vi "Graphic_UI_Main.vi"(7 "Graphic UI Exit":refnum<user-event>, 11 "manager_daemon":refnum<class "manager_daemon.lvclass">) -> ()   [LabVIEW 2024]
uses:
  typedefs/volume.type.colors--cluster.ctl
  comic_manager/manager_daemon/manager_daemon.lvclass
  <vilib>/Utility/miscctls.llb/LVPositionTypeDef.ctl
  <vilib>/Utility/miscctls.llb/LVPoint32TypeDef.ctl
  CV_Shared_Library/volume.object--cluster.ctl
  CV_Shared_Library/volume.type--enum.ctl
  comic_manager/TypeDefs/issue.display--cluster.ctl
  typedefs/picture.data--cluster.ctl
  typedefs/filters--cluster.ctl
  comic_manager/manager_daemon/manager_daemon.lvclass/manager_daemon.ctl
  comic_manager/TypeDefs/graphic.filter--cluster.ctl
  <vilib>/addons/_JKI Toolkits/State Machine/_JKI_lib_State_Machine.llb/Select State(s)_err__jki_lib_state_machine.vi
  <vilib>/addons/_JKI Toolkits/State Machine/_JKI_lib_State_Machine.llb/Periodic Trigger__ogtk__JKI-SM__jki_lib_state_machine.vi
  CV_Shared_Library/CV_Shared_Library.lvlib
panel:
  in  "change volume types":bool
  in  "dest type":T1=enum."Reprint/Document" caption="Enum"
  in  "source type":T1=enum."One Shot" caption="Enum"
  in  "search string":string
  in  "publisher":u16(ring)
  in  "advanced filter":bool
  in  "Release Week":timestamp format="%<%x>T"
  out "filter dates":cluster{"start":timestamp, "end":timestamp}={"start"=timestamp(3328668000 s since 1904-01-01), "end"=timestamp(3785292000 s since 1904-01-01)} {"start" format="%<%x>T"; "end" format="%<%x>T"}
  in  "zoom filter":bool
  in  "generate report":bool
  in  "Show/Hide Issues":bool
  in  "clear title":bool
  in  "titles":string[](array[string])=["x-men"]
  in  "Show All Comics":bool
  in  "Volume Type":T2={"Ongoing"=TRUE, "Limited Series"=TRUE, "Annuals"=TRUE, "One Shots"=TRUE, "Reference/Reprints"=TRUE, "Digital"=TRUE}
  in  "Exit":bool
  in  "Legend":T3={"ongoing"=34559, "Limited Series"=35193, "Annuals"=16754450, "One Shots"=7566195, "Reprints"=16722176, "Digital"=49407}
  out "2D Picture":picture
  in  "Show Legend":bool=TRUE
  in  "Step Size":enum32{"Monthly", "Yearly"}(radio)
  in  "inc time":bool
  in  "dec time":bool
  in  "dec end":bool
  in  "dec start":bool
  in  "inc start":bool
  in  "inc end":bool
  in  "Plot End":timestamp=timestamp(3785292000 s since 1904-01-01) format="%<%x>T"
  in  "Plot Start":timestamp=timestamp(3318732000 s since 1904-01-01) format="%<%x>T"
  out "volume":string="uncanny x-men (1981)"
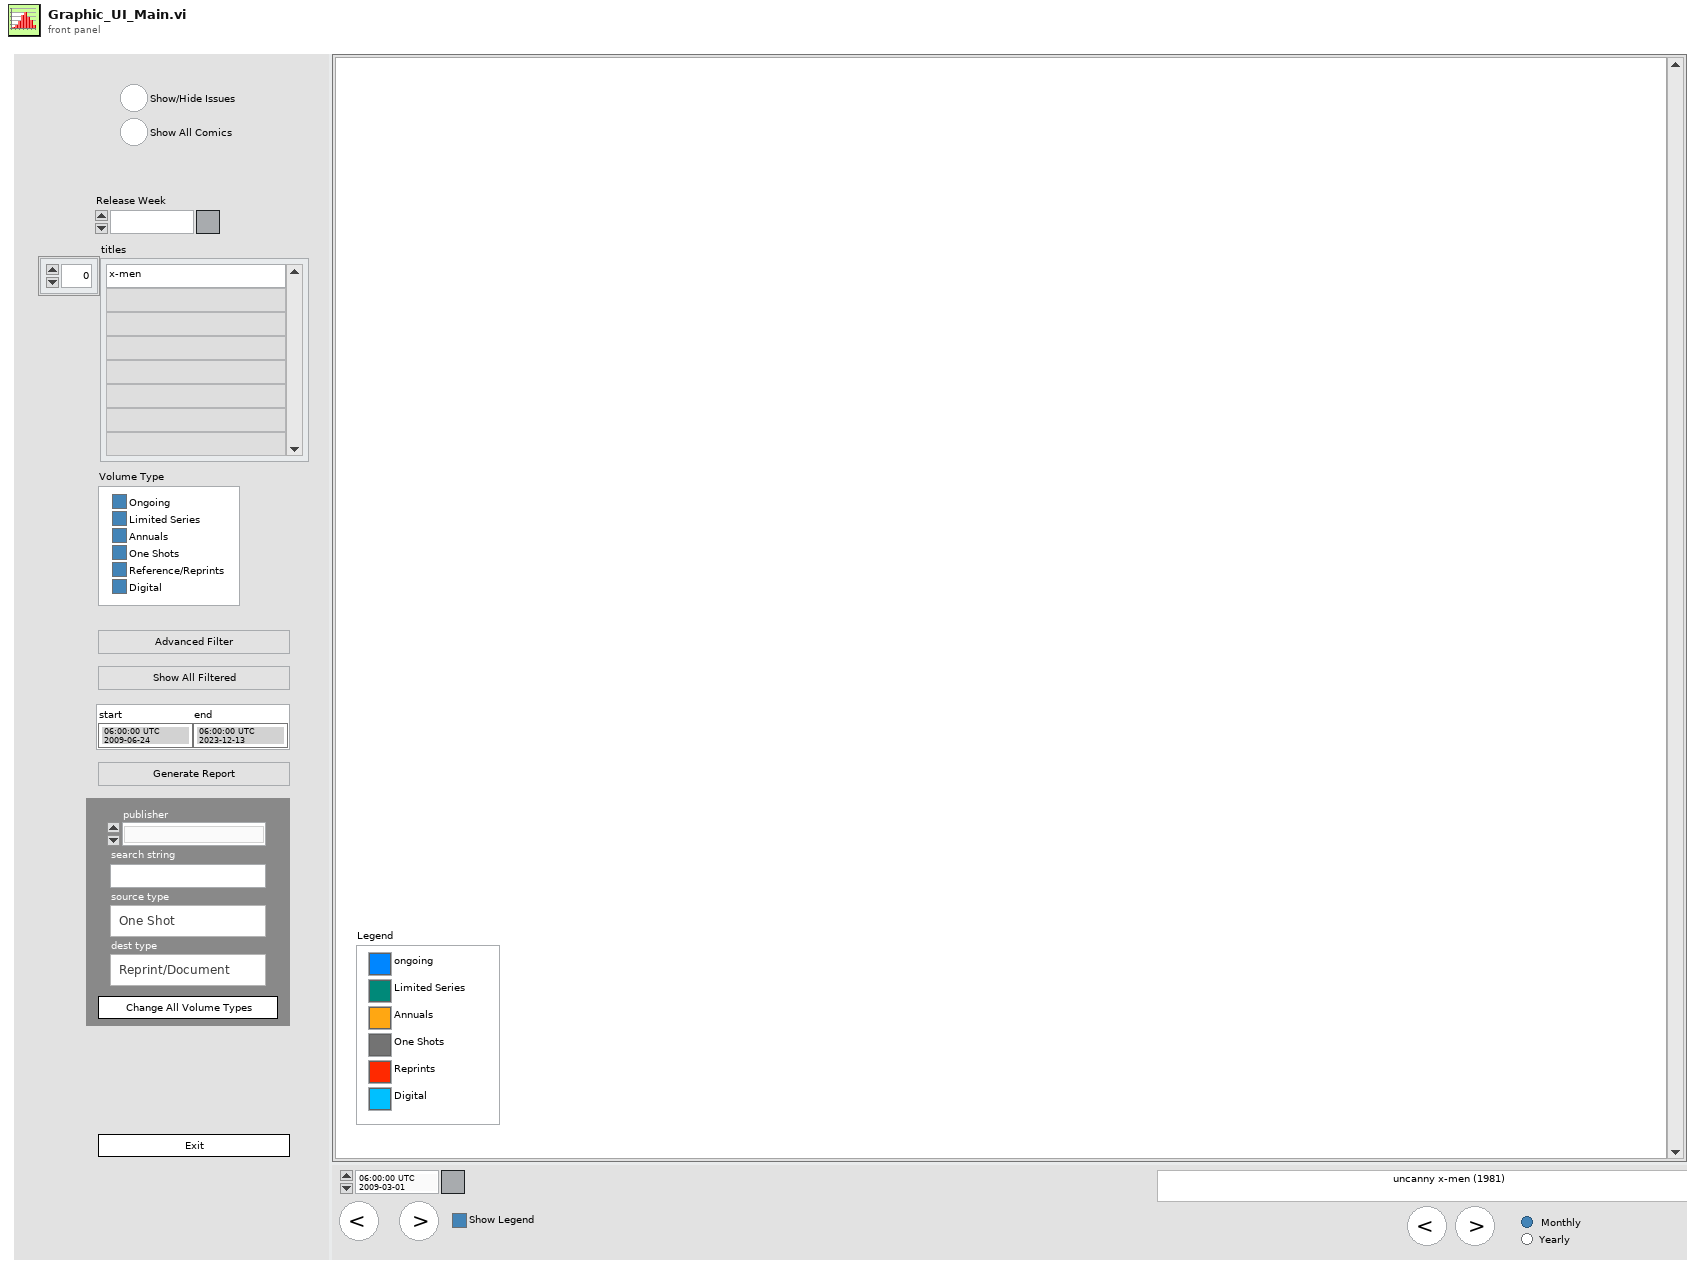
[diagram p1: front panel]
types:
  T1 = typedef "CV_Shared_Library.lvlib/volume.type--enum.ctl" = enum16{"Ongoing", "Limited Series", "Annual", "One Shot", "Reprint/Document", "Digital"}
  T2 = cluster{"Ongoing":bool, "Limited Series":bool, "Annuals":bool, "One Shots":bool, "Reference/Reprints":bool, "Digital":bool}
  T3 = typedef "volume.type.colors--cluster.ctl" = cluster{"ongoing":u32, "Limited Series":u32, "Annuals":u32, "One Shots":u32, "Reprints":u32, "Digital":u32}
  T4 = cluster{"search string":string, "source type":T1, "dest type":T1, "publisher":string}
  T5 = enum8{"Enabled", "Disabled", "Disabled and Grayed Out"}
  T6 = typedef "LVPositionTypeDef.ctl" = cluster{"Left":i32, "Top":i32}
  T7 = enum32{"Invalid", "Standard", "Closed", "Hidden", "Minimized", "Maximized"}
  T8 = enum32{"invalid app kind", "Development System", "Run Time System", "Student Edition", "Embedded LabVIEW", "Evaluation", "Custom"}
  T9 = typedef "filters--cluster.ctl" = cluster{"team filter":string[], "story filter":string[], "char filter":string[], "concept filter":string[], "Apply Filters":enum32{"AND", "OR"}}
  T10 = typedef "CV_Shared_Library.lvlib/graphic.filter--cluster.ctl" = cluster{"Volume Type":cluster{"Ongoing":bool, "Limited Series":bool, "Annuals":bool, "One Shots":bool, "Reference/Reprints":bool, "Digital":bool}, "team":string[], "characters":string[], "storyArcs":string[], "Plot End":timestamp, "Plot Start":timestamp, "title":string[], "colors":T3, "concept":string[], "show all":bool, "Search by Title":enum32{"AND", "OR"}, "pub ids":i32[]}
  T11 = cluster{"left":i16, "top":i16, "right":i16, "bottom":i16}
  T12 = typedef "CV_Shared_Library.lvlib/volume.object--cluster.ctl" = cluster{"start date":timestamp, "end date":timestamp, "sortable_name":string, "color":u32, "volume type":T1, "issues":T13[]}
  T13 = typedef "CV_Shared_Library.lvlib/issue.display--cluster.ctl" = cluster{"cover_date":timestamp, "id":i32, "number":string, "fill":bool, "hilight":bool}
  T14 = typedef "picture.data--cluster.ctl" = cluster{"names":string[], "colors":u32[], "cells":cluster{"left":i16, "top":i16, "right":i16, "bottom":i16}[], "end date":timestamp, "start date":timestamp}
  T15 = typedef "LVPoint32TypeDef.ctl" = cluster{"Horizontal":i32, "Vertical":i32}
  T16 = cluster{"Core":cluster{"Current VI Reference":refnum<vi>, "Close Panel on Exit?":bool}, "volume objects":cluster{"Array":T12[]}[], "picture data":T14, "picture":picture, "rows":cluster{"left":i16, "top":i16, "right":i16, "bottom":i16}[], "cursor":T15, "manager_daemon":refnum<class "manager_daemon.lvclass">, "filter dates":cluster{"start":timestamp, "end":timestamp}, "filters":T9, "pub filter event":refnum<user-event>, "pub ids":i32[], "filter event":refnum<user-event>, "Graphic UI Exit":refnum<user-event>, "filter exit":refnum<user-event>}
  T17 = typedef "manager_daemon.lvclass/PublisherMap--map.ctl" = map{string, T18}
  T18 = typedef "manager_daemon.lvclass/PublisherData--cluster.ctl" = cluster{"id":i32, "volumes":set{i32}}
  T19 = cluster{"left":i16, "top":i16, "right":i16, "bottom":i16}[]
  T20 = cluster{"Current VI Reference":refnum<vi>, "Close Panel on Exit?":bool}
  T21 = cluster{"filter data event":refnum<user-event>, "search titles event":refnum<user-event>}
  T22 = typedef "LVBoundsTypeDef.ctl" = cluster{"Width":u32, "Height":u32}
  T23 = typedef "LVPointTypeDef.ctl" = cluster{"Horizontal":i16, "Vertical":i16}
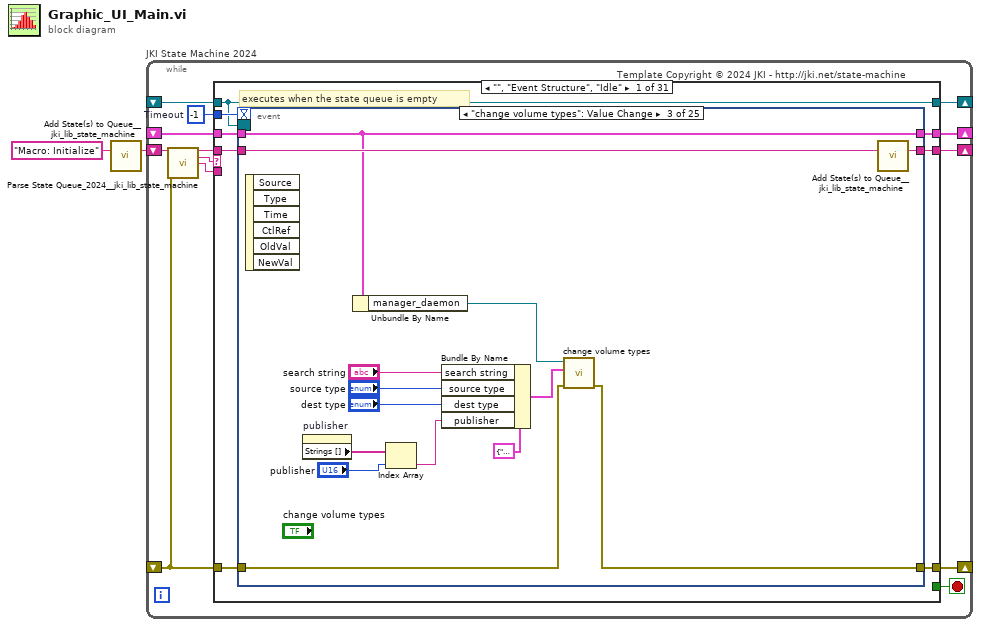
[diagram p0: block diagram]
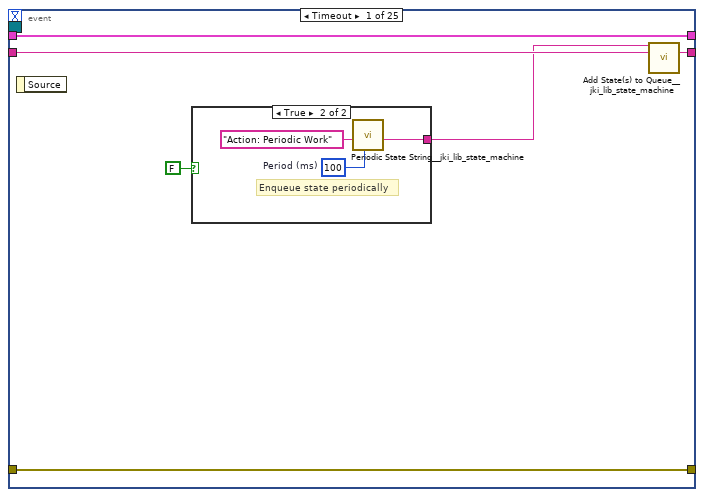
[diagram p2: hidden frame]
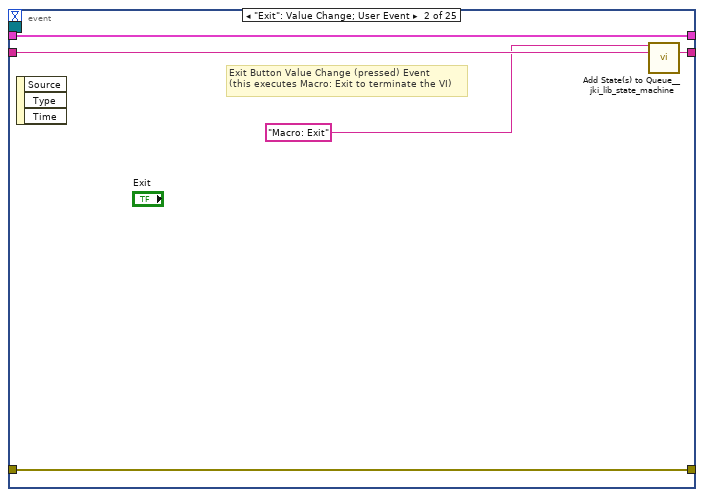
[diagram p4: hidden frame]
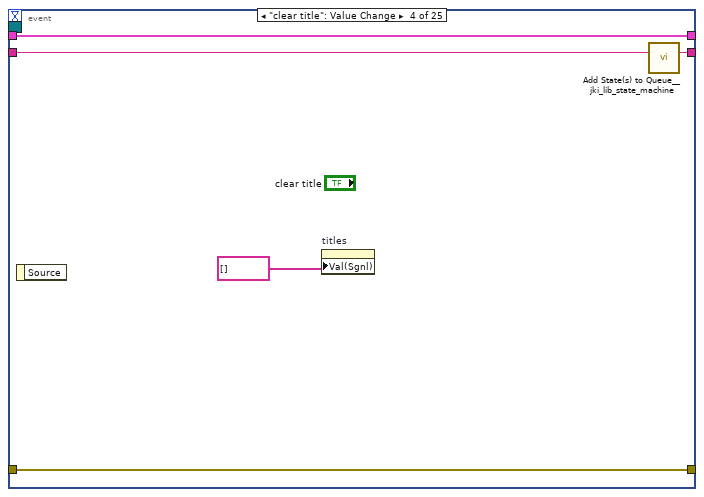
[diagram p5: hidden frame]
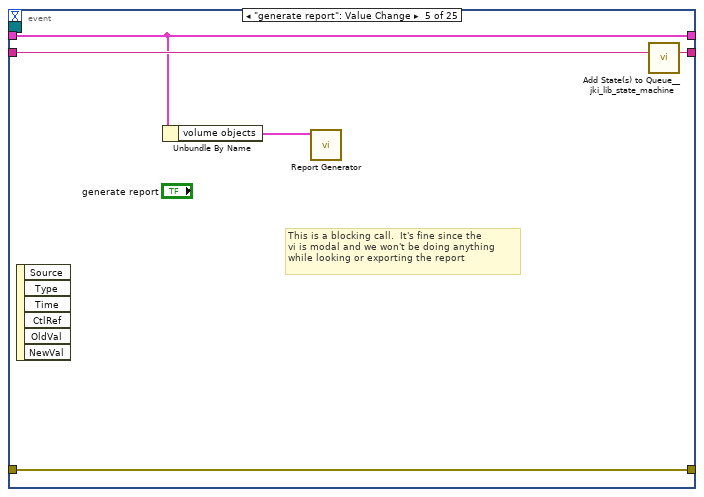
[diagram p6: hidden frame]
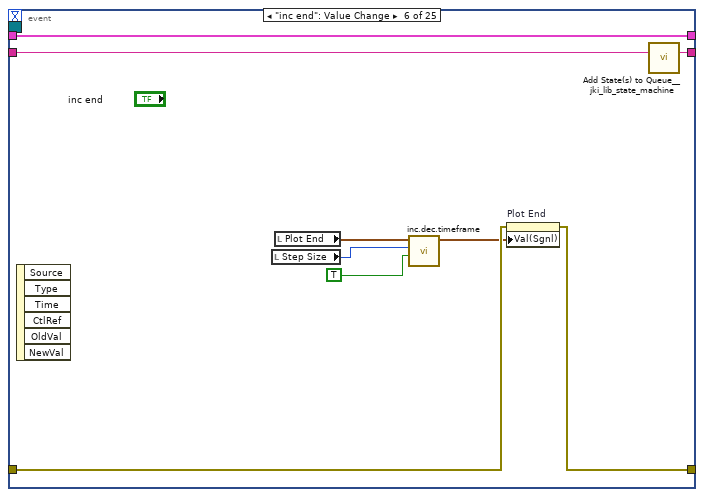
[diagram p7: hidden frame]
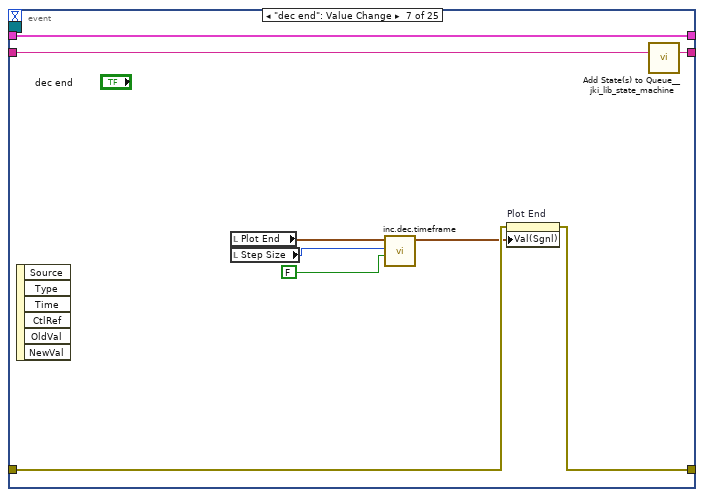
[diagram p8: hidden frame]
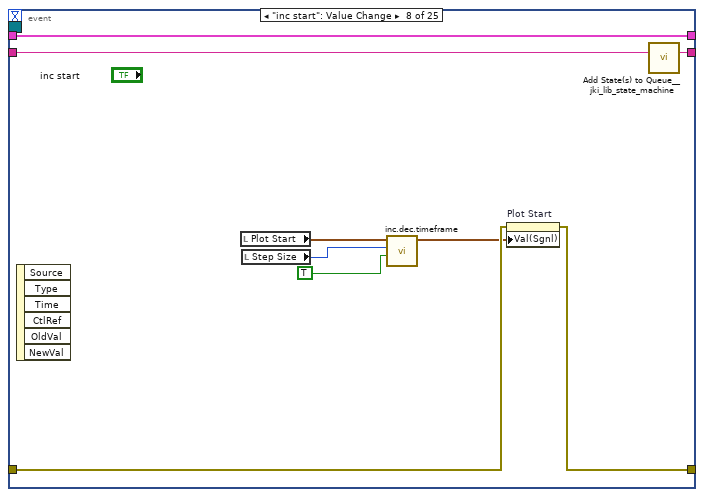
[diagram p9: hidden frame]
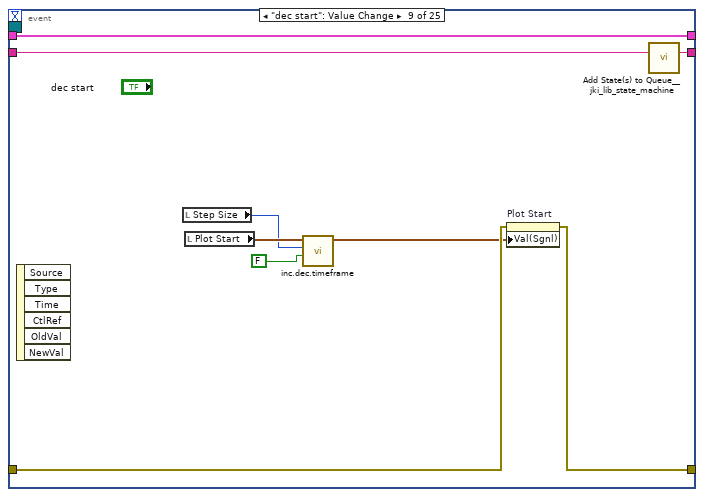
[diagram p10: hidden frame]
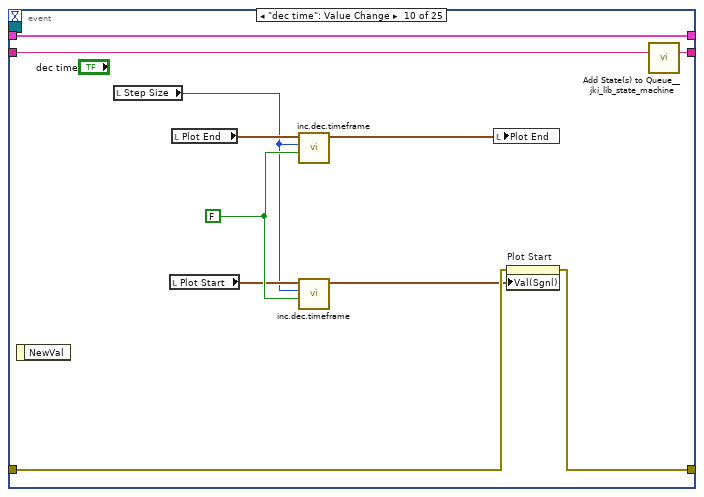
[diagram p11: hidden frame]
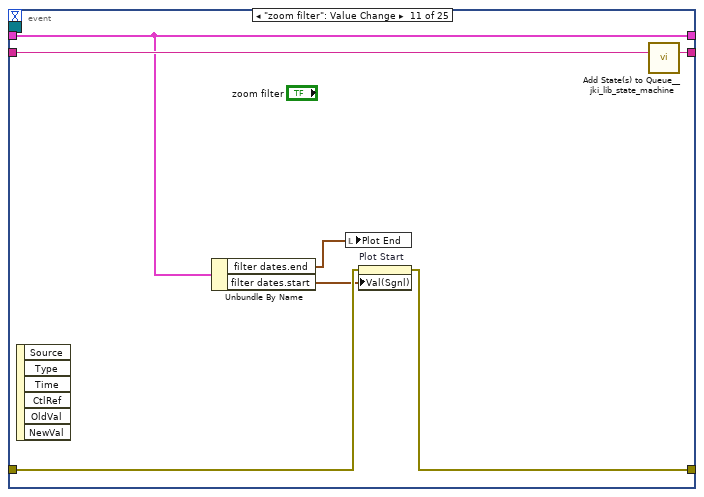
[diagram p12: hidden frame]
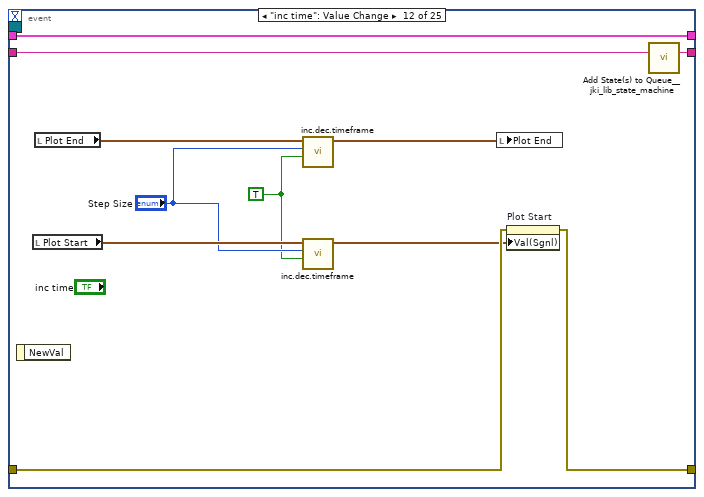
[diagram p13: hidden frame]
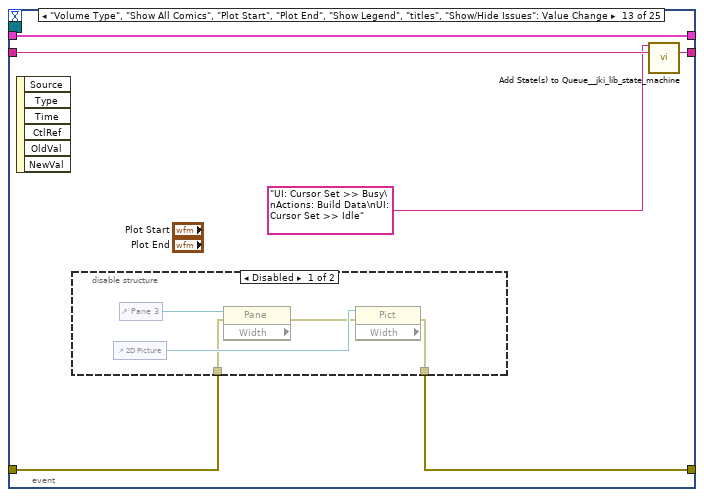
[diagram p14: hidden frame]
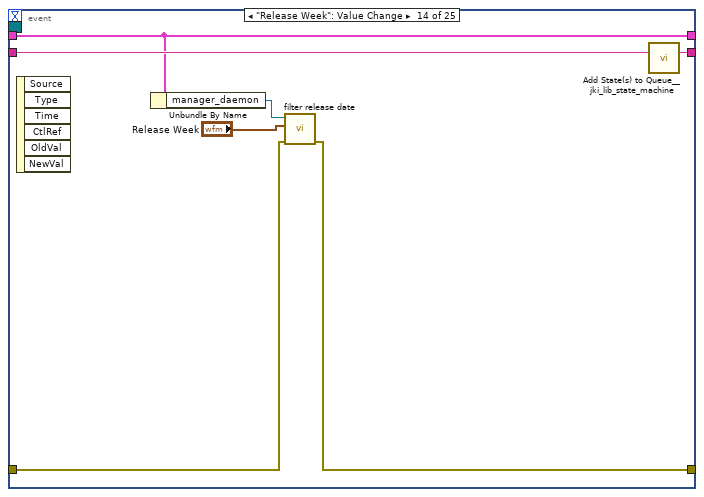
[diagram p16: hidden frame]
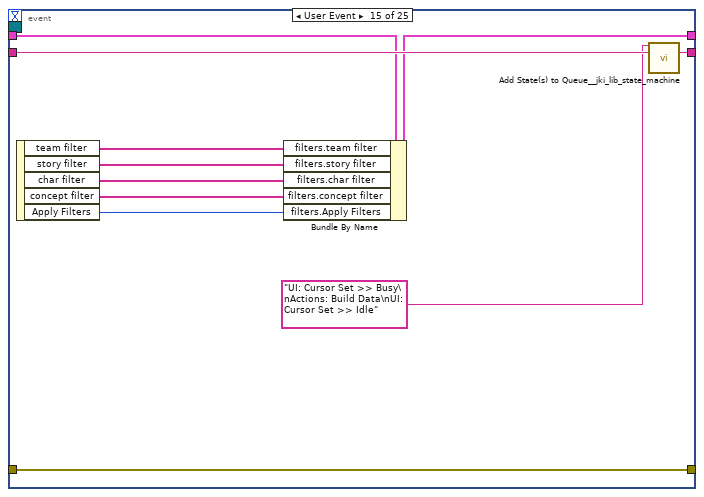
[diagram p17: hidden frame]
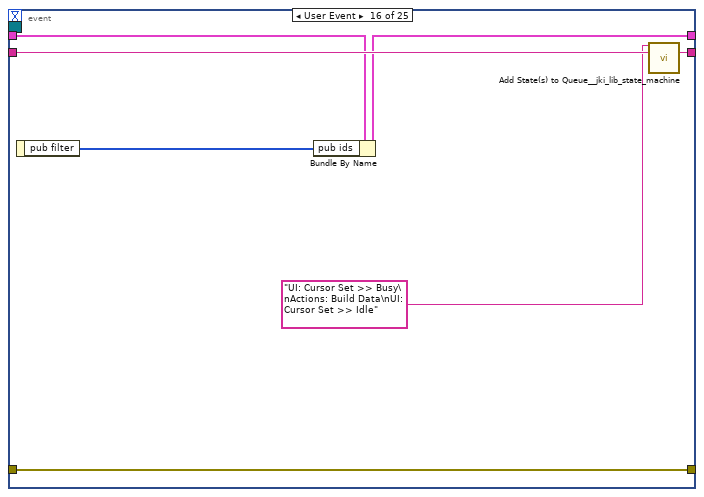
[diagram p18: hidden frame]
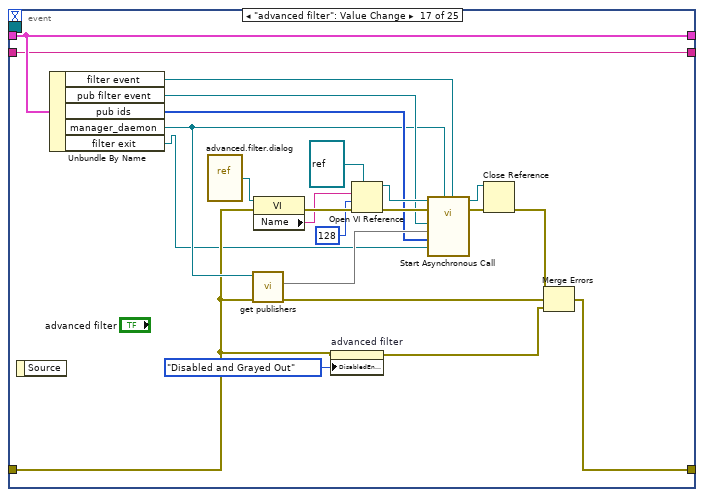
[diagram p19: hidden frame]
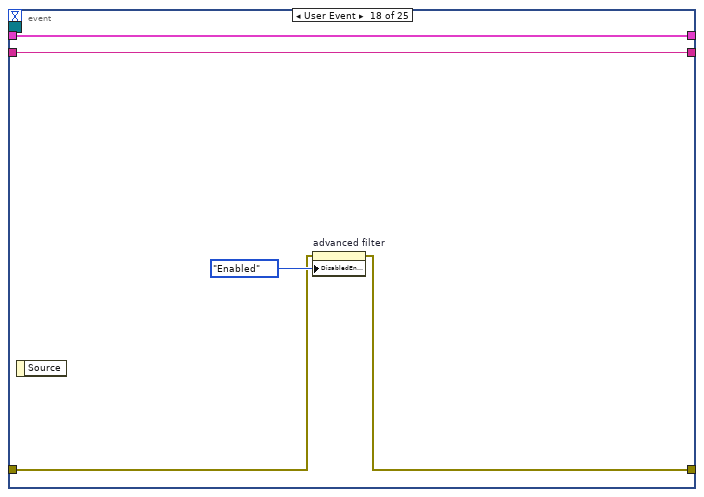
[diagram p20: hidden frame]
diagram:
  n1 = call <vilib>:"Add State(s) to Queue__jki_lib_state_machine.vi"("State(s) in (\"\")"="Macro: Initialize") -> ("States Out"=w2:string)  [unwired: 14 in]
  n2 = while "JKI State Machine 2024" {
    shift-right: [w8] -> _
    shift-left: _ -> [w7]
    shift-right: [w11] -> _
    shift-left: _ -> [w5]
    shift-right: [w10] -> _
    shift-left: w2 -> [w12]
    shift-right: [w4] -> _
    shift-left: _ -> [w3]
    stop <- w9 stop-if-true
    w6 = -1  # Timeout
    # "Template Copyright © 2024 JKI - http://jki.net/state-machine"
    n3 = call <vilib>:"Parse State Queue_2024__jki_lib_state_machine.vi"("State Queue"=w12, "Error In (no error)"=w5) -> ("Remaining States"=w14:string, "Current State"=w15:string, "Arguments"=w13:string)  [unwired: 11 in]
    n4 = case shown="\"\", \"Event Structure\", \"Idle\"" w15 {
      selector: w15 -> [_ _ w290 _ _ _ _ _ _ _ _ _ _ _ _ _ _ _ _ _ _ _ _ _ _ _ _ _ _ _ _]
      tunnel: w14 -> [w23 w288 w294 w314 w325 w335 w340 w359 w384 w389 w409 w415 w420 w430 w446 w454 w459 w466 w478 w548 w554 w564 w569 w579 w590 w602 w614 w633 w655 w669 w693]
      tunnel: w13 -> [_ _ _ _ w320 _ _ _ _ _ _ _ _ _ w442 _ _ w461 w472 _ _ _ _ _ _ _ _ _ _ _ _]
      tunnel: w7 -> [w21 w285 w292 w307 w322 w333 w337 _ w381 w386 w403 w413 w417 w427 w441 w452 w457 w464 w474 w545 w551 w562 w566 w573 w588 w600 w611 w631 w646 w663 w685]
      tunnel: [w20 w286 w296 w311 errorcluster {"status"=FALSE, "code"=0, "source"=""} ("error out") w332 w338 w356 w379 w387 w407 w410 w418 w421 w434 w451 w456 w462 w475 w546 w552 w559 w567 w571 w585 w597 w612 w628 w645 w667 w692] -> w11
      tunnel: w5 -> [w17 w286 w295 w311 w321 w332 w338 w356 w374 w387 w393 w411 w418 w425 w433 w451 w456 w463 w476 w546 w552 w559 w567 w575 w587 w599 w612 w629 w644 w667 w692]
      tunnel: [w22 w287 w293 w313 w324 w334 w339 w358 w383 w388 w408 w414 w419 w429 w445 w453 w458 w465 w477 w547 w553 w563 w568 w578 w589 w601 w613 w632 w654 w668 w693] -> w10
      tunnel: [_ _ _ _ _ TRUE _ _ _ _ _ _ _ _ _ _ _ _ _ _ _ _ _ _ _ _ _ _ _ _ _] -> w9
      tunnel: [w19 w285 w292 w312 w322 w333 w337 w357 w381 w386 w401 w413 w417 w427 w441 w452 w457 w464 w474 w545 w551 w562 w566 w570 w588 w595 w611 w631 w646 w662 w684] -> w8
      tunnel: w6 -> [w18 _ _ _ _ _ _ _ _ _ _ _ _ _ _ _ _ _ _ _ _ _ _ _ _ _ _ _ _ _ _]
      tunnel: [w16 w284 w289 w301 w315 w330 w336 w349 w380 w385 w394 w412 w416 w428 w444 w450 w455 w460 w471 w544 w549 w555 w565 w577 w582 w592 w603 w627 w648 w660 w680] -> w4
      tunnel: w3 -> [w16 w284 w289 w301 w315 w330 w336 w349 w380 w385 _ w412 w416 w428 w444 w450 w455 w460 w471 w544 w549 w555 w565 w577 w582 w592 w603 w627 w648 w660 w680]
      frame "", "Event Structure", "Idle" {
        # "executes when the state queue is empty"
        n5 = event shown="[2] \"change volume types\": Value Change" {
          selector: w16 -> [_ _ _ _ _ _ _ _ _ _ _ _ _ _ _ _ _ _ _ _ _ _ _ _ _]
          dyn-events: _ -> [_ _ _ _ _ _ _ _ _ _ _ _ _ _ _ _ _ _ _ _ _ _ _ _ _]
          timeout: w18 -> [_ _ _ _ _ _ _ _ _ _ _ _ _ _ _ _ _ _ _ _ _ _ _ _ _]
          tunnel: w23 -> [w29 w37 w51 w56 w61 w70 w79 w88 w97 w108 w115 w126 w132 w145 w156 w163 w177 w190 w201 w225 w229 w246 w263 w271 w283]
          tunnel: [w28 w36 w50 w55 w60 w69 w78 w87 w96 w107 w114 w125 w131 w144 w155 w162 w177 w190 w200 w224 w229 w245 w262 w270 w282] -> w22
          tunnel: w21 -> [w26 w34 w39 w53 w58 w68 w77 w86 w95 w106 w111 w124 w129 w143 w152 w159 w179 w191 w202 w222 w230 w244 w252 w268 w280]
          tunnel: [w27 w35 w48 w54 w59 w66 w75 w84 w93 w104 w112 w122 w127 w140 w154 w161 w170 w187 w199 w205 w226 w231 w261 w267 w281] -> w20
          tunnel: w17 -> [w27 w35 w49 w54 w59 w67 w76 w85 w94 w105 w113 w123 w128 w139 w154 w161 w167 w188 w199 w206 w227 w242 w261 w266 w281]
          tunnel: [w26 w34 w39 w53 w58 w68 w77 w86 w95 w106 w111 w124 w129 w143 w151 w158 w179 w191 w202 w221 w230 w244 w251 w268 w280] -> w19
          event Timeout {
            n6 = event-data() -> ()  [unwired: 1 in, 1 out]
            n7 = case shown="True" FALSE {
              tunnel: [_ w32] -> w25
              frame False {
              }
              frame True {
                w30 = u32 100  # Period (ms)
                # "Enqueue state periodically"
                n8 = call <vilib>:"Periodic State String__jki_lib_state_machine.vi"("Period (ms)"=w30, "State"="Action: Periodic Work") -> ("State Out"=w32:string)  [unwired: 9 in]
              }
            }
            n9 = call <vilib>:"Add State(s) to Queue__jki_lib_state_machine.vi"("State(s) in Front (\"\")"=w25, "State(s) in (\"\")"=w29) -> ("States Out"=w28:string)  [unwired: 13 in]
          }
          event "Exit": Value Change; User Event {
            # "Exit Button Value Change (pressed) Event\n(this executes Macro: Exit to terminate the VI)"
            n10 = event-data() -> ()  [unwired: 1 in, 3 out]
            n11 = call <vilib>:"Add State(s) to Queue__jki_lib_state_machine.vi"("State(s) in Front (\"\")"="Macro: Exit", "State(s) in (\"\")"=w37) -> ("States Out"=w36:string)  [unwired: 13 in]
          }
          event "change volume types": Value Change {
            n12 = event-data() -> ()  [unwired: 1 in, 6 out]
            n13 = property on="publisher" class="Ring (strict)"() -> ("Strings []"=w43:string[])  [unwired: 2 in, 2 out]
            n14 = Unbundle By Name(w39) -> ("manager_daemon"=w38:refnum<class "manager_daemon.lvclass">)
            n15 = Index Array(array=w43, index="publisher") -> (element=w41:string)
            n16 = Bundle By Name(cluster=T4 {"search string"="", "source type"=enum."Ongoing", "dest type"=enum."Ongoing", "publisher"=""} ("change criteria"), "search string"="search string", "source type"="source type", "dest type"="dest type", "publisher"=w41) -> (w40:T4)
            n17 = call "change volume types.vi"("error in (no error)"=w49, "change criteria"=w40, "manager_daemon in"=w38) -> ("error out"=w48:errorcluster)  [unwired: 7 in, 1 out]
            n18 = call <vilib>:"Add State(s) to Queue__jki_lib_state_machine.vi"("State(s) in (\"\")"=w51) -> ("States Out"=w50:string)  [unwired: 14 in]
          }
          event "clear title": Value Change {
            n19 = event-data() -> ()  [unwired: 1 in, 1 out]
            n20 = property on="titles" class="Arr (strict)"("Val(Sgnl)"=string[] []) -> ()  [unwired: 2 in, 2 out]
            n21 = call <vilib>:"Add State(s) to Queue__jki_lib_state_machine.vi"("State(s) in (\"\")"=w56) -> ("States Out"=w55:string)  [unwired: 14 in]
          }
          event "generate report": Value Change {
            # "This is a blocking call.  It's fine since the \nvi is modal and we won't be doing anything\nwhile looking or exporting the report"
            n22 = event-data() -> ()  [unwired: 1 in, 6 out]
            n23 = Unbundle By Name(w58) -> ("volume objects"=w57:cluster{"Array":T12[]}[])
            n24 = call "Report Generator.vi"("volume objects"=w57) -> ()  [unwired: 11 in]
            n25 = call <vilib>:"Add State(s) to Queue__jki_lib_state_machine.vi"("State(s) in (\"\")"=w61) -> ("States Out"=w60:string)  [unwired: 14 in]
          }
          event "inc end": Value Change {
            n26 = event-data() -> ()  [unwired: 1 in, 6 out]
            n27 = local read "Step Size"() -> (w63:enum32{"Monthly", "Yearly"})
            n28 = local read "Plot End"() -> (w65:timestamp)
            n29 = call "inc.dec.timeframe.vi"("inc (T)"=TRUE, "Step Size"=w63, "Plot End"=w65) -> ("time stamp"=w64:timestamp)  [unwired: 8 in]
            n30 = property on="Plot End" class="AbsTime (strict)"(error in=w67, "Val(Sgnl)"=w64) -> (error out=w66:errorcluster)  [unwired: 1 in, 1 out]
            n31 = call <vilib>:"Add State(s) to Queue__jki_lib_state_machine.vi"("State(s) in (\"\")"=w70) -> ("States Out"=w69:string)  [unwired: 14 in]
          }
          event "dec end": Value Change {
            n32 = event-data() -> ()  [unwired: 1 in, 6 out]
            n33 = local read "Plot End"() -> (w74:timestamp)
            n34 = local read "Step Size"() -> (w72:enum32{"Monthly", "Yearly"})
            n35 = call "inc.dec.timeframe.vi"("inc (T)"=FALSE, "Step Size"=w72, "Plot End"=w74) -> ("time stamp"=w73:timestamp)  [unwired: 8 in]
            n36 = property on="Plot End" class="AbsTime (strict)"(error in=w76, "Val(Sgnl)"=w73) -> (error out=w75:errorcluster)  [unwired: 1 in, 1 out]
            n37 = call <vilib>:"Add State(s) to Queue__jki_lib_state_machine.vi"("State(s) in (\"\")"=w79) -> ("States Out"=w78:string)  [unwired: 14 in]
          }
          event "inc start": Value Change {
            n38 = event-data() -> ()  [unwired: 1 in, 6 out]
            n39 = local read "Plot Start"() -> (w83:timestamp)
            n40 = local read "Step Size"() -> (w81:enum32{"Monthly", "Yearly"})
            n41 = call "inc.dec.timeframe.vi"("inc (T)"=TRUE, "Step Size"=w81, "Plot End"=w83) -> ("time stamp"=w82:timestamp)  [unwired: 8 in]
            n42 = property on="Plot Start" class="AbsTime (strict)"(error in=w85, "Val(Sgnl)"=w82) -> (error out=w84:errorcluster)  [unwired: 1 in, 1 out]
            n43 = call <vilib>:"Add State(s) to Queue__jki_lib_state_machine.vi"("State(s) in (\"\")"=w88) -> ("States Out"=w87:string)  [unwired: 14 in]
          }
          event "dec start": Value Change {
            n44 = event-data() -> ()  [unwired: 1 in, 6 out]
            n45 = local read "Step Size"() -> (w90:enum32{"Monthly", "Yearly"})
            n46 = local read "Plot Start"() -> (w92:timestamp)
            n47 = call "inc.dec.timeframe.vi"("inc (T)"=FALSE, "Step Size"=w90, "Plot End"=w92) -> ("time stamp"=w91:timestamp)  [unwired: 8 in]
            n48 = property on="Plot Start" class="AbsTime (strict)"(error in=w94, "Val(Sgnl)"=w91) -> (error out=w93:errorcluster)  [unwired: 1 in, 1 out]
            n49 = call <vilib>:"Add State(s) to Queue__jki_lib_state_machine.vi"("State(s) in (\"\")"=w97) -> ("States Out"=w96:string)  [unwired: 14 in]
          }
          event "dec time": Value Change {
            w101 = FALSE ("inc (T)")
            n50 = event-data() -> ()  [unwired: 1 in, 1 out]
            n51 = local read "Step Size"() -> (w98:enum32{"Monthly", "Yearly"})
            n52 = local read "Plot Start"() -> (w100:timestamp)
            n53 = local read "Plot End"() -> (w103:timestamp)
            n54 = call "inc.dec.timeframe.vi"("inc (T)"=w101, "Step Size"=w98, "Plot End"=w103) -> ("time stamp"=w102:timestamp)  [unwired: 8 in]
            n55 = call "inc.dec.timeframe.vi"("inc (T)"=w101, "Step Size"=w98, "Plot End"=w100) -> ("time stamp"=w99:timestamp)  [unwired: 8 in]
            n56 = local write "Plot End"(w102) -> ()
            n57 = property on="Plot Start" class="AbsTime (strict)"(error in=w105, "Val(Sgnl)"=w99) -> (error out=w104:errorcluster)  [unwired: 1 in, 1 out]
            n58 = call <vilib>:"Add State(s) to Queue__jki_lib_state_machine.vi"("State(s) in (\"\")"=w108) -> ("States Out"=w107:string)  [unwired: 14 in]
          }
          event "zoom filter": Value Change {
            n59 = event-data() -> ()  [unwired: 1 in, 6 out]
            n60 = Unbundle By Name(w111) -> ("filter dates.end"=w109:timestamp, "filter dates.start"=w110:timestamp)
            n61 = local write "Plot End"(w109) -> ()
            n62 = property on="Plot Start" class="AbsTime (strict)"(error in=w113, "Val(Sgnl)"=w110) -> (error out=w112:errorcluster)  [unwired: 1 in, 1 out]
            n63 = call <vilib>:"Add State(s) to Queue__jki_lib_state_machine.vi"("State(s) in (\"\")"=w115) -> ("States Out"=w114:string)  [unwired: 14 in]
          }
          event "inc time": Value Change {
            w116 = TRUE ("inc (T)")
            n64 = event-data() -> ()  [unwired: 1 in, 1 out]
            n65 = local read "Plot Start"() -> (w119:timestamp)
            n66 = local read "Plot End"() -> (w121:timestamp)
            n67 = call "inc.dec.timeframe.vi"("inc (T)"=w116, "Step Size"="Step Size", "Plot End"=w121) -> ("time stamp"=w120:timestamp)  [unwired: 8 in]
            n68 = call "inc.dec.timeframe.vi"("inc (T)"=w116, "Step Size"="Step Size", "Plot End"=w119) -> ("time stamp"=w118:timestamp)  [unwired: 8 in]
            n69 = local write "Plot End"(w120) -> ()
            n70 = property on="Plot Start" class="AbsTime (strict)"(error in=w123, "Val(Sgnl)"=w118) -> (error out=w122:errorcluster)  [unwired: 1 in, 1 out]
            n71 = call <vilib>:"Add State(s) to Queue__jki_lib_state_machine.vi"("State(s) in (\"\")"=w126) -> ("States Out"=w125:string)  [unwired: 14 in]
          }
          event "Volume Type", "Show All Comics", "Plot Start", "Plot End", "Show Legend", "titles", "Show/Hide Issues": Value Change {
            n72 = event-data() -> ()  [unwired: 1 in, 6 out]
            n73 = disable-structure shown="Disabled" {
              disable-tunnel: w128 -> [w134 w138]
              disable-tunnel: [w133 w138] -> w127
              frame Disabled {
                n74 = control-ref of="2D Picture"() -> (w136:refnum<vi>)
                n75 = control-ref of="Pane 3"() -> (w137:refnum<vi>)
                n76 = property class="Pane" props=["Width"](reference=w137, error in=w134) -> (error out=w135:errorcluster)  [unwired: 2 out]
                n77 = property class="Pict" props=["Width"](reference=w136, error in=w135) -> (error out=w133:errorcluster)  [unwired: 2 out]
              }
              frame Enabled {
              }
            }
            n78 = call <vilib>:"Add State(s) to Queue__jki_lib_state_machine.vi"("State(s) in Front (\"\")"="UI: Cursor Set >> Busy\nActions: Build Data\nUI: Cursor Set >> Idle", "State(s) in (\"\")"=w132) -> ("States Out"=w131:string)  [unwired: 13 in]
          }
          event "Release Week": Value Change {
            n79 = event-data() -> ()  [unwired: 1 in, 6 out]
            n80 = Unbundle By Name(w143) -> ("manager_daemon"=w142:refnum<class "manager_daemon.lvclass">)
            n81 = call "filter release date.vi"("error in (no error)"=w139, "Release Week"="Release Week", "manager_daemon in"=w142) -> ("error out"=w140:errorcluster)  [unwired: 7 in, 1 out]
            n82 = call <vilib>:"Add State(s) to Queue__jki_lib_state_machine.vi"("State(s) in (\"\")"=w145) -> ("States Out"=w144:string)  [unwired: 14 in]
          }
          event User Event {
            n83 = event-data() -> ("team filter"=w150:string[], "story filter"=w149:string[], "char filter"=w148:string[], "concept filter"=w147:string[], "Apply Filters"=w146:enum32{"AND", "OR"})  [unwired: 1 in]
            n84 = Bundle By Name(cluster=w152, "filters.team filter"=w150, "filters.story filter"=w149, "filters.char filter"=w148, "filters.concept filter"=w147, "filters.Apply Filters"=w146) -> (w151:T16)
            n85 = call <vilib>:"Add State(s) to Queue__jki_lib_state_machine.vi"("State(s) in Front (\"\")"="UI: Cursor Set >> Busy\nActions: Build Data\nUI: Cursor Set >> Idle", "State(s) in (\"\")"=w156) -> ("States Out"=w155:string)  [unwired: 13 in]
          }
          event User Event {
            n86 = event-data() -> ("pub filter"=w157:i32[])  [unwired: 1 in]
            n87 = Bundle By Name(cluster=w159, "pub ids"=w157) -> (w158:T16)
            n88 = call <vilib>:"Add State(s) to Queue__jki_lib_state_machine.vi"("State(s) in Front (\"\")"="UI: Cursor Set >> Busy\nActions: Build Data\nUI: Cursor Set >> Idle", "State(s) in (\"\")"=w163) -> ("States Out"=w162:string)  [unwired: 13 in]
          }
          event "advanced filter": Value Change {
            n89 = event-data() -> ()  [unwired: 1 in, 1 out]
            n90 = Unbundle By Name(w179) -> ("filter event"=w168:refnum<user-event>, "pub filter event"=w178:refnum<user-event>, "pub ids"=w173:i32[], "manager_daemon"=w169:refnum<class "manager_daemon.lvclass">, "filter exit"=w164:refnum<user-event>)
            n91 = vi-ref "advanced.filter.dialog.vi"() -> (w186:refnum<vi>)
            n92 = call "get publishers.vi"("error in (no error)"=w167, "manager_daemon in"=w169) -> ("error out"=w171:errorcluster, "Publisher Map"=w174:T17)  [unwired: 7 in, 1 out]
            n93 = property class="VI"(reference=w186, error in=w167) -> (error out=w185:errorcluster, "Name"=w183:string)  [unwired: 1 out]
            n94 = property on="advanced filter" class="Bool"(error in=w167, "DisabledEnum"=T5."Disabled and Grayed Out" ("Disabled")) -> (error out=w166:errorcluster)  [unwired: 1 in, 1 out]
            n95 = Open VI Reference(type specifier VI Refnum (for type only)=refnum<vi> refnum, vi path=w183, options=128, error in (no error)=w185) -> (vi reference=w180:refnum<vi>, error out=w181:errorcluster)  [unwired: 2 in]
            n96 = call-by-ref "Start Asynchronous Call"(reference=w180, error in=w181, "filters events"=w168, "manager_daemon"=w169, "filter exit event"=w164, "filtered publisher ids"=w173, "map"=w174, "pub filter event"=w178) -> (reference out=w175:refnum<vi>, error out=w176:errorcluster)  [unwired: 6 in]
            n97 = Close Reference(reference=w175, error in (no error)=w176) -> (error out=w172:errorcluster)
            n98 = Merge Errors(w172, w171, w166) -> (w170:errorcluster)
          }
          event User Event {
            n99 = event-data() -> ()  [unwired: 1 in, 1 out]
            n100 = property on="advanced filter" class="Bool"(error in=w188, "DisabledEnum"=T5."Enabled" ("Disabled")) -> (error out=w187:errorcluster)  [unwired: 1 in, 1 out]
          }
          event "2D Picture": Mouse Wheel {
            n101 = event-data() -> ("Orientation"=w198:enum16{"Horizontal", "Vertical"})  [unwired: 1 in]
            n102 = property on="2D Picture" class="Pict"() -> ("Top"=w196:i16)  [unwired: 2 in, 2 out]
            n103 = Equal?(x=w198, y=enum16{"Horizontal", "Vertical"}."Vertical") -> (x = y?=w195:bool)
            n104 = Greater Or Equal To 0?(x=w196) -> (x >= 0?=w194:bool)
            n105 = And(x=w195, y=w194) -> (x .and. y?=w193:bool)
            n106 = case shown="False" w193 {
              tunnel: [_ "UI: Cursor Set >> Busy\nActions: Build Data\nUI: Cursor Set >> Idle"] -> w192
              frame False {
                n107 = property on="2D Picture" class="Pict"("Top"=i16 0 ("Origin:Top")) -> ()  [unwired: 2 in, 2 out]
              }
              frame True {
              }
            }
            n108 = call <vilib>:"Add State(s) to Queue__jki_lib_state_machine.vi"("State(s) in Front (\"\")"=w192, "State(s) in (\"\")"=w201) -> ("States Out"=w200:string)  [unwired: 13 in]
          }
          event User Event {
            w213 = timestamp(0 s since 1904-01-01)
            n109 = event-data() -> ("filtered data"=w217:T12[], "filter dates"=w216:cluster{"start":timestamp, "end":timestamp})  [unwired: 1 in]
            "filter dates" <- w216
            n110 = Unbundle(w216) -> ("start"=w215:timestamp, "end"=w214:timestamp)
            n111 = Equal?(x=w213, y=w215) -> (x = y?=w212:bool)
            n112 = Equal?(x=w214, y=w213) -> (x = y?=w211:bool)
            n113 = call "sort.volumes.vi"("volumes"=w217) -> ("end date"=w218:timestamp, "start date"=w219:timestamp, "volumes by row"=w220:cluster{"Array":T12[]}[])  [unwired: 8 in]
            n114 = Or(x=w212, y=w211) -> (x .or. y?=w210:bool)
            n115 = Select(t=T5."Disabled and Grayed Out" ("Disabled"), s=w210, f=T5."Enabled" ("Disabled")) -> (s? t:f=w207:T5)
            n116 = Bundle By Name(cluster=w222, "volume objects"=w220, "picture data.start date"=w219, "picture data.end date"=w218, "filter dates"=w216) -> (w221:T16)
            n117 = property on="zoom filter" class="Bool"(error in=w206, "DisabledEnum"=w207) -> (error out=w205:errorcluster)  [unwired: 1 in, 1 out]
            n118 = call <vilib>:"Add State(s) to Queue__jki_lib_state_machine.vi"("State(s) in Front (\"\")"="UI: Cursor Set >> Busy\nUI: FP Update >> TRUE\nActions: Calculate Rows\nActions: Draw Grid\nActions: Calculate Cells\nActions: Draw Picture\nUI: FP Update >> FALSE\nUI: Cursor Set >> Idle", "State(s) in (\"\")"=w225) -> ("States Out"=w224:string)  [unwired: 13 in]
          }
          event User Event {
            n119 = event-data() -> ("titles"=w228:string[])  [unwired: 1 in]
            n120 = property on="titles" class="Arr (strict)"(error in=w227, "Val(Sgnl)"=w228) -> (error out=w226:errorcluster)  [unwired: 1 in, 1 out]
          }
          event Panel Resize {
            n121 = event-data() -> ("VIRef"=w243:refnum<vi>)  [unwired: 1 in]
            n122 = call "resize.navigation.pane.vi"("error in (no error)"=w242, "vi ref"=w243) -> ("error out"=w240:errorcluster)  [unwired: 9 in]
            n123 = invoke on="2D Picture" class="Pict" method="FitControlToPane"(error in=w240) -> (error out=w239:errorcluster)  [unwired: 2 in, 2 out]
            n124 = property on="2D Picture" class="Pict"(error in=w239) -> (error out=w232:errorcluster, "Height"=w236:u32)  [unwired: 1 in, 1 out]
            n125 = Subtract(x=w236, y=u32 259) -> (x-y=w234:u32)
            n126 = Bundle By Name(cluster=T6 {"Left"=0, "Top"=0} ("Position"), "Top"=w234, "Left"=24) -> (w233:T6)
            n127 = property on="Legend" class="Clust (strict)"(error in=w232, "Position"=w233) -> (error out=w231:errorcluster)  [unwired: 1 in, 1 out]
            n128 = call <vilib>:"Add State(s) to Queue__jki_lib_state_machine.vi"("State(s) in Front (\"\")"="UI: Cursor Set >> Busy\nActions: Build Data\nUI: Cursor Set >> Idle", "State(s) in (\"\")"=w246) -> ("States Out"=w245:string)  [unwired: 13 in]
          }
          event "2D Picture": Mouse Move {
            n129 = event-data() -> ("Coords"=w255:T15)  [unwired: 1 in]
            n130 = property on="2D Picture" class="Pict"() -> ("Position"=w260:T6, "Top"=w247:i16)  [unwired: 2 in, 2 out]
            n131 = Unbundle By Name(w255) -> ("Horizontal"=w259:i32, "Vertical"=w257:i32)
            n132 = Unbundle By Name(w260) -> ("Left"=w258:i32, "Top"=w256:i32)
            n133 = Subtract(x=w259, y=w258) -> (x-y=w254:i32)
            n134 = Subtract(x=w257, y=w256) -> (x-y=w249:i32)
            n135 = Add(x=w249, y=w247) -> (x+y=w248:i32)
            n136 = Bundle By Name(cluster=w255, "Horizontal"=w254, "Vertical"=w248) -> (w250:T15)
            n137 = Bundle By Name(cluster=w252, "cursor"=w250) -> (w251:T16)
            n138 = call <vilib>:"Add State(s) to Queue__jki_lib_state_machine.vi"("State(s) in Front (\"\")"="Actions: Display Cursor" ("State(s) in Front (\"\")"), "State(s) in (\"\")"=w263) -> ("States Out"=w262:string)  [unwired: 13 in]
          }
          event "2D Picture": Mouse Down? {
            n139 = event-data() -> ("Coords"=w269:T15, "Mods.Double Click"=w264:bool)  [unwired: 1 in]
            n140 = case shown="True" w264 {
              tunnel: w269 -> [_ _]
              tunnel: w268 -> [_ w277]
              tunnel: w266 -> [w272 w274]
              tunnel: [w272 w273] -> w267
              frame False {
              }
              frame True {
                n141 = Unbundle By Name(w277) -> ("manager_daemon"=w276:refnum<class "manager_daemon.lvclass">)
                n142 = local read "volume"() -> (w275:string)
                n143 = call "display info.vi"("error in (no error)"=w274, "volume name"=w275, "manager_daemon in"=w276) -> ("error out"=w273:errorcluster)  [unwired: 7 in, 1 out]
              }
            }
            n144 = event-data("Discard?"=TRUE) -> ()  [unwired: 4 in, 1 out]
            n145 = call <vilib>:"Add State(s) to Queue__jki_lib_state_machine.vi"("State(s) in (\"\")"=w271) -> ("States Out"=w270:string)  [unwired: 14 in]
          }
          event Panel Close? {
            # "Discard the event because we'll close the front panel ourselves in Macro: Exit"
            # "Close Panel button (pressed) Event\n(this executes Macro: Exit to terminate the VI)"
            n146 = event-data() -> ()  [unwired: 1 in, 1 out]
            n147 = event-data("Discard?"=TRUE) -> ()  [unwired: 1 in, 1 out]
            n148 = call <vilib>:"Add State(s) to Queue__jki_lib_state_machine.vi"("State(s) in Front (\"\")"="Macro: Exit", "State(s) in (\"\")"=w283) -> ("States Out"=w282:string)  [unwired: 13 in]
          }
        }
      }
      frame "---------- Core ----------" {
        # "Do not put any code in this frame.\n(it is a separator no-op)"
        n149 = call <vilib>:"Add State(s) to Queue__jki_lib_state_machine.vi"("State(s) in (\"\")"=w288) -> ("States Out"=w287:string)  [unwired: 14 in]
      }
      frame Default {
        w299 = 42 items=["No error", "Argument error", "Memory is full", "Out of zone", "End of file", "File already open", "Generic file I/O error", "File not found", "File permission error", "Disk is full", "Duplicate path", "Too many files open", "System feature not enabled", "Resource file not found", "Cannot add resource", "Resource not found", "Image not found", "Image memory error", "Pen does not exist", "Config type invalid", "Config token not found", "Config parse error", "Config memory error", "Bad external code format", "Bad external code offset", "External code not present", "Null window", "Destroy window error", "Null menu", "Print aborted", "Bad print record", "Print driver error", "Windows error during printing", "Memory error during printing", "Print dialog error", "Generic print error", "Invalid device refnum", "Device not found", "Device parameter error", "Device unit error", "Cannot open device", "Device call aborted", "Generic error", "Cancelled by user", "Object ID too low", "Object ID too high", "Object not in heap", "Unknown heap", "Unknown object (invalid DefProc)", "Unknown object (DefProc not in table)", "Message out of range", "Invalid (null) method", "Unknown message", "Manager call not supported", "Bad address", "Network operation in progress", "Network operation timed out", "Connection is busy", "Network attribute not supported", "Network error", "Address in use", "System out of memory", "Connection aborted", "Connection refused", "Not connected", "Already connected", "Connection closed", "Initialization error (interapplication manager)", "Bad occurrence", "Wait on unbound occurrence handler", "Occurrence queue overflow", "Datalog type conflict", "Unused", "Unrecognized type (interapplication manager)", "Memory corrupt", "Failed to make temporary DLL", "Old CIN version", "Drag socket not found", "Failed to load drop-object", "Failed to register OLE object", "Failed to release OLE object", "Format specifier type mismatch", "Unknown format specifier", "Too few format specifiers", "Too many format specifiers", "Scan failed", "Newer CIN version", "Error converting to variant", "Runtime menu error", "Password tampered", "Variant attribute not found", "Incompatible variant data type", "Event data is not available", "Event Store is not present", "Occurrence is not found", "Event Queue is not created", "Event info is not available", "Refnum passed is NULL", "Error retrieving Class GUID", "Error retrieving CoClass GUID", "Error retrieving TypeLib GUID.", "Bad built application magic bytes.", "Specific driver is different from the specific driver associated with the Logical Name.", "There is no session opened to the class driver.", "Max Error", "MAX - Error with config objects", "MAX - Error loading configuration", "MAX - Group not supported"]
        # "Current State"
        # "Do not delete, rename, or modify this frame.\n(this is used to capture unhandled states and typos)"
        # "Handle mistyped state name (developer tool)"
        n150 = Format Into String(format string="Software Exception: Unhandled State \"%s\"." ("message"), error in=w295, w290) -> (resulting string=w298:string, error out=w297:errorcluster)  [unwired: 1 in]
        n151 = call <vilib>:"Error Cluster From Error Code.vi"("show call chain? (False)"=TRUE, "error in (no error)"=w297, "error message (\"\")"=w298, "error code (0)"=w299) -> ("error out"=w296:errorcluster)  [unwired: 5 in]
        n152 = call <vilib>:"Add State(s) to Queue__jki_lib_state_machine.vi"("State(s) in (\"\")"=w294) -> ("States Out"=w293:string)  [unwired: 14 in]
      }
      frame "Initialize Core Data" {
        # "Do not delete, rename, or modify this frame.\n(this is used to determine panel behavior on exit)"
        # "originally closed?"
        # "exe?"
        # "If panel starts closed or is an EXE, then close it when we exit"
        n153 = property class="VI"() -> ("FP.State"=w304:T7)  [unwired: 2 in, 2 out]
        n154 = property class="App"() -> ("App.Kind"=w310:T8)  [unwired: 2 in, 2 out]
        n155 = control-ref of="Current VI Reference"() -> (w305:refnum<vi>)
        n156 = Equal?(x=w304, y=T7."Closed" ("Front Panel Window:State")) -> (x = y?=w302:bool)
        n157 = Equal?(x=w310, y=T8."Run Time System" ("Application:Kind")) -> (x = y?=w308:bool)
        n158 = Or(x=w302, y=w308) -> (x .or. y?=w306:bool)
        n159 = Bundle By Name(cluster=w307, "Core.Current VI Reference"=w305, "Core.Close Panel on Exit?"=w306) -> (w312:T16)
        n160 = call <vilib>:"Add State(s) to Queue__jki_lib_state_machine.vi"("State(s) in (\"\")"=w314) -> ("States Out"=w313:string)  [unwired: 14 in]
      }
      frame "Error Handler" {
        # "When running as sourcecode, this function will add previous state data to the error message to aid the developer in troubleshoot errors.\nIf run as an executable, no additional information is added to the error message."
        # "This state receives both Errors and Warnings which is how the Status of this wire can be FALSE"
        # "Unhandled Error -- Display it"
        # "Handle any errors or warnings here.\nYou can also output any states to clean-up after errors or warnings occur"
        # "Clear error or warning"
        n161 = disable-structure shown="Default" {
          disable-tunnel: w321 -> [w328 w329]
          disable-tunnel: w320 -> [w327 _]
          disable-tunnel: [w326 w329] -> w319
          frame condition #0 (active) {
            n162 = call <vilib>:"Append Error Details__jki_lib_state_machine.vi"("error in (no error)"=w328, "Previous State and Argument(s)"=w327) -> ("error out"=w326:errorcluster)  [unwired: 9 in]
          }
          frame condition #1 {
          }
        }
        n163 = call <vilib>:"General Error Handler.vi"("error in (no error)"=w319) -> ()  [unwired: 10 in, 5 out]
        n164 = call-poly <vilib>:"Select State(s)__jki_lib_state_machine.vi"("State(s) if True (\"\")"="/* Post Error States", "Select"=w319, "State(s) if False (\"\")"="/* Post Warning States") -> ("States Out"=w317:string)  [unwired: 12 in]
        n165 = call <vilib>:"Add State(s) to Queue__jki_lib_state_machine.vi"("State(s) in Front (\"\")"=w317, "State(s) in (\"\")"=w325) -> ("States Out"=w324:string)  [unwired: 13 in]
      }
      frame "Exit" {
        # "Do not put any code in this frame.\n(No errors that occur here will be handled.)"
        n166 = call <vilib>:"Add State(s) to Queue__jki_lib_state_machine.vi"("State(s) in (\"\")"=w335) -> ("States Out"=w334:string)  [unwired: 14 in]
      }
      frame "---------- Data ----------" {
        # "Do not put any code in this frame.\n(It is a separator no-op. You can make a copy of this frame to create a new Data frame)"
        n167 = call <vilib>:"Add State(s) to Queue__jki_lib_state_machine.vi"("State(s) in (\"\")"=w340) -> ("States Out"=w339:string)  [unwired: 14 in]
      }
      frame "Data: Initialize" {
        w341 = refnum<user-event> refnum  # filter exit
        w343 = T9 {"team filter"=[], "story filter"=[], "char filter"=[], "concept filter"=[], "Apply Filters"=enum."AND"}  # filters
        w344 = refnum<user-event> refnum  # filter event
        w345 = i32[] []  # pub ids
        w346 = refnum<user-event> refnum  # pub filter event
        w347 = cluster{"start":timestamp, "end":timestamp} {"start"=timestamp(0 s since 1904-01-01), "end"=timestamp(0 s since 1904-01-01)}  # filter dates
        w350 = T14 {"names"=[], "colors"=[], "cells"=[], "end date"=timestamp(0 s since 1904-01-01), "start date"=timestamp(0 s since 1904-01-01)}  # picture data
        w351 = cluster{"Array":T12[]}[] []  # volume objects
        w352 = T15 {"Horizontal"=0, "Vertical"=0}  # cursor
        w353 = T19 []  # rows
        w354 = picture data[5B]  # picture
        w355 = T20 {"Current VI Reference"=refnum, "Close Panel on Exit?"=FALSE}  # Core
        # "Data names and types of shift register data are defined by this bundle."
        # "Initialize the shift-register data, here.\n(data names are defined by what you wire into the bundle function)"
        n168 = Bundle("Core"=w355, "volume objects"=w351, "picture data"=w350, "picture"=w354, "rows"=w353, "cursor"=w352, "manager_daemon"="manager_daemon", "filter dates"=w347, "filters"=w343, "pub filter event"=w346, "pub ids"=w345, "filter event"=w344, "Graphic UI Exit"="Graphic UI Exit", "filter exit"=w341) -> (w357:T16)  [unwired: 1 in]
        n169 = call <vilib>:"Add State(s) to Queue__jki_lib_state_machine.vi"("State(s) in (\"\")"=w359) -> ("States Out"=w358:string)  [unwired: 14 in]
      }
      frame "Data: Cleanup" {
        # "Cleanup any data and references, here.\n(this is called automatically, by the Macro: Exit)"
        n170 = Unbundle By Name(w381) -> ("filter event"=w375:refnum<user-event>, "pub filter event"=w377:refnum<user-event>, "Core.Current VI Reference"=w382:refnum<vi>, "Graphic UI Exit"=w372:refnum<user-event>, "filter exit"=w364:refnum<user-event>)
        n171 = Generate User Event(user event=w372, event data cluster=TRUE ("event data")) -> (error out=w370:errorcluster)  [unwired: 2 in, 1 out]
        n172 = Generate User Event(user event=w364, event data cluster=TRUE ("event data")) -> (user event out=w363:refnum<user-event>, error out=w366:errorcluster)  [unwired: 2 in]
        n173 = Close Reference(reference=w382) -> (error out=w378:errorcluster)  [unwired: 1 in]
        n174 = call <vilib>:"Clear Errors.vi"("error in (no error)"=w370, "specific error code to clear (0: all)"=1) -> ("error out"=w368:errorcluster)  [unwired: 4 in, 1 out]
        n175 = call <vilib>:"Clear Errors.vi"("error in (no error)"=w366, "specific error code to clear (0: all)"=1) -> ("error out"=w362:errorcluster)  [unwired: 4 in, 1 out]
        n176 = Destroy User Event(user event=w377) -> (error out=w376:errorcluster)  [unwired: 1 in]
        n177 = Destroy User Event(user event=w375) -> (error out=w373:errorcluster)  [unwired: 1 in]
        n178 = Destroy User Event(user event=w363, error in=w362) -> (error out=w361:errorcluster)
        n179 = call <vilib>:"Clear Errors.vi"("error in (no error)"=w361) -> ("error out"=w360:errorcluster)  [unwired: 5 in, 1 out]
        n180 = Merge Errors(w374, w373, w376, w378, w368, w360) -> (w379:errorcluster)
        n181 = call <vilib>:"Add State(s) to Queue__jki_lib_state_machine.vi"("State(s) in (\"\")"=w384) -> ("States Out"=w383:string)  [unwired: 14 in]
      }
      frame "---------- Events ----------" {
        # "Do not put any code in this frame.\n(It is a separator no-op. You can make a copy of this frame to create a new UI frame)"
        n182 = call <vilib>:"Add State(s) to Queue__jki_lib_state_machine.vi"("State(s) in (\"\")"=w389) -> ("States Out"=w388:string)  [unwired: 14 in]
      }
      frame "Events: Register" {
        w392 = FALSE  # filter exit
        w404 = i32[] []  # pub filter
        n183 = Unbundle By Name(w403) -> ("manager_daemon"=w406:refnum<class "manager_daemon.lvclass">, "Graphic UI Exit"=w395:refnum<user-event>)
        n184 = Create User Event(user event datatype=T9 {"team filter"=[], "story filter"=[], "char filter"=[], "concept filter"=[], "Apply Filters"=enum."AND"} ("filters")) -> (user event=w397:refnum<user-event>, error out=w399:errorcluster)  [unwired: 1 in]
        n185 = Create User Event(user event datatype=w404, error in=w393) -> (user event=w402:refnum<user-event>, error out=w400:errorcluster)
        n186 = Create User Event(user event datatype=w392, error in=w393) -> (user event=w390:refnum<user-event>, error out=w391:errorcluster)
        n187 = call "GraphicUI.events.get.vi"("manager_daemon in"=w406) -> ("graphic ui events"=w405:T21)  [unwired: 9 in, 1 out]
        n188 = Merge Errors(w399, w400, w391) -> (w398:errorcluster)
        n189 = Bundle By Name(cluster=w403, "filter event"=w397, "pub filter event"=w402, "filter exit"=w390) -> (w401:T16)
        n190 = register-events(error in=w398, w397, w402, w405, w395, w390) -> (reference out=w394:refnum<event-registration>, error out=w407:errorcluster)  [unwired: 1 in]
        n191 = call <vilib>:"Add State(s) to Queue__jki_lib_state_machine.vi"("State(s) in (\"\")"=w409) -> ("States Out"=w408:string)  [unwired: 14 in]
      }
      frame "Events: Unregister" {
        # "Do not put any code in this frame.\n(It is a separator no-op. You can make a copy of this frame to create a new UI frame)"
        n192 = Unregister For Events(event registration refnum=w412, error in=w411) -> (error out=w410:errorcluster)
        n193 = call <vilib>:"Add State(s) to Queue__jki_lib_state_machine.vi"("State(s) in (\"\")"=w415) -> ("States Out"=w414:string)  [unwired: 14 in]
      }
      frame "---------- UI ----------" {
        n194 = call <vilib>:"Add State(s) to Queue__jki_lib_state_machine.vi"("State(s) in (\"\")"=w420) -> ("States Out"=w419:string)  [unwired: 14 in]
      }
      frame "UI: Populate Publishers" {
        n195 = Unbundle By Name(w427) -> ("manager_daemon"=w426:refnum<class "manager_daemon.lvclass">)
        n196 = call "get publishers.vi"("error in (no error)"=w425, "manager_daemon in"=w426) -> ("error out"=w423:errorcluster, "Publisher Map"=w424:T17)  [unwired: 7 in, 1 out]
        n197 = for {
          tunnel: w424 -> [w432] mode=indexing
          tunnel: [w431] -> w422 mode=indexing
          n198 = Unbundle By Name(w432) -> ("name"=w431:string)
        }
        n199 = property on="publisher" class="Ring (strict)"(error in=w423, "Strings []"=w422) -> (error out=w421:errorcluster)  [unwired: 1 in, 1 out]
        n200 = call <vilib>:"Add State(s) to Queue__jki_lib_state_machine.vi"("State(s) in (\"\")"=w430) -> ("States Out"=w429:string)  [unwired: 14 in]
      }
      frame "UI: FP Update" {
        n201 = Equal?(x=w442, y="TRUE") -> (x = y?=w438:bool)
        n202 = Unbundle By Name(w441) -> ("Core.Current VI Reference"=w440:refnum<vi>)
        n203 = property class="VI"(reference=w440, error in=w433) -> (error out=w437:errorcluster, "Panel"=w439:refnum<vi>)  [unwired: 1 out]
        n204 = property class="Pnl"(reference=w439, error in=w437, "DeferPanUpdts"=w438) -> (reference out=w435:refnum<vi>, error out=w436:errorcluster)
        n205 = Close Reference(reference=w435, error in (no error)=w436) -> (error out=w434:errorcluster)
        n206 = call <vilib>:"Add State(s) to Queue__jki_lib_state_machine.vi"("State(s) in (\"\")"=w446) -> ("States Out"=w445:string)  [unwired: 14 in]
      }
      frame "UI: Initialize" {
        # "Initialize the User Interface, here.\n(this is called automatically, by the Macro: Initialize)"
        n207 = Get Date/Time In Seconds() -> (seconds since 1Jan1904=w449:timestamp)
        n208 = local write "Show All Comics"(FALSE) -> ()
        n209 = local write "Release Week"(w449) -> ()
        n210 = property on="advanced filter" class="Bool"("DisabledEnum"=T5."Enabled" ("Disabled")) -> ()  [unwired: 2 in, 2 out]
        n211 = call <vilib>:"Add State(s) to Queue__jki_lib_state_machine.vi"("State(s) in (\"\")"=w454) -> ("States Out"=w453:string)  [unwired: 14 in]
      }
      frame "UI: Uninitialize" {
        # "Cleanup the User Interface, here.\n(this is called automatically, by the Macro: Exit)"
        n212 = call <vilib>:"Add State(s) to Queue__jki_lib_state_machine.vi"("State(s) in (\"\")"=w459) -> ("States Out"=w458:string)  [unwired: 14 in]
      }
      frame "UI: Cursor Set" {
        # "Argument"
        # "Set and Unset Cursor Busy.\n(Usage: \"UI: Cursor Set >> Busy|Idle\")"
        n213 = case shown="\"Busy\"" w461 {
          tunnel: w463 -> [w468 w470]
          tunnel: [w467 w469] -> w462
          frame "Idle", Default {
            n214 = call <vilib>:"Unset Busy.vi"("error in (no error)"=w468) -> ("error out"=w467:errorcluster)  [unwired: 10 in]
          }
          frame "Busy" {
            n215 = call <vilib>:"Set Busy.vi"("error in (no error)"=w470) -> ("error out"=w469:errorcluster)  [unwired: 9 in, 1 out]
          }
        }
        n216 = call <vilib>:"Add State(s) to Queue__jki_lib_state_machine.vi"("State(s) in (\"\")"=w466) -> ("States Out"=w465:string)  [unwired: 14 in]
      }
      frame "UI: Front Panel State" {
        # "Argument"
        # "Set Front Panel Open or Closed\n(Usage: \"UI: Front Panel State >> Open|Close\")"
        n217 = Unbundle By Name(w474) -> ("Core.Current VI Reference"=w473:refnum<vi>)
        n218 = case shown="\"Minimize\", \"Minimized\"" w472 {
          tunnel: w476 -> [w484 w499 w510 w523 w536]
          tunnel: [w486 w500 w512 w525 w538] -> w475
          tunnel: w473 -> [w485 w497 w511 w524 w537]
          frame "Open", "Standard", Default {
            w479 = T7."Standard" ("State")
            n219 = property class="VI"(reference=w485, error in=w484) -> (reference out=w482:refnum<vi>, error out=w483:errorcluster, "FP.State"=w481:T7)
            n220 = Not Equal?(x=w481, y=w479) -> (x != y?=w480:bool)
            n221 = case shown="True" w480 {
              tunnel: [w490 w492] -> w486
              tunnel: w483 -> [w489 w492]
              tunnel: w482 -> [w488 _]
              tunnel: w479 -> [w487 _]
              frame True {
                n222 = invoke class="VI" method="FP.Open"(reference=w488, error in=w489, "Activate"=TRUE, "State"=w487) -> (error out=w490:errorcluster)  [unwired: 1 in, 4 out]
              }
              frame False {
              }
            }
          }
          frame "Close", "Closed" {
            n223 = property class="VI"(reference=w497, error in=w499) -> (reference out=w496:refnum<vi>, error out=w498:errorcluster, "FP.State"=w494:T7)
            n224 = Not Equal?(x=w494, y=T7."Closed" ("Front Panel Window:State")) -> (x != y?=w493:bool)
            n225 = case shown="True" w493 {
              tunnel: [w501 w504] -> w500
              tunnel: w498 -> [w501 w503]
              tunnel: w496 -> [_ w502]
              frame False {
              }
              frame True {
                n226 = invoke class="VI" method="FP.Close"(reference=w502, error in=w503) -> (error out=w504:errorcluster)  [unwired: 1 in, 2 out]
              }
            }
          }
          frame "Hidden", "Hide" {
            w505 = T7."Hidden" ("State")
            n227 = property class="VI"(reference=w511, error in=w510) -> (reference out=w508:refnum<vi>, error out=w509:errorcluster, "FP.State"=w507:T7)
            n228 = Not Equal?(x=w507, y=w505) -> (x != y?=w506:bool)
            n229 = case shown="True" w506 {
              tunnel: [w516 w517] -> w512
              tunnel: w509 -> [w515 w517]
              tunnel: w508 -> [w514 _]
              tunnel: w505 -> [w513 _]
              frame True {
                n230 = invoke class="VI" method="FP.Open"(reference=w514, error in=w515, "State"=w513) -> (error out=w516:errorcluster)  [unwired: 2 in, 4 out]
              }
              frame False {
              }
            }
          }
          frame "Minimize", "Minimized" {
            w518 = T7."Minimized" ("State")
            n231 = property class="VI"(reference=w524, error in=w523) -> (reference out=w521:refnum<vi>, error out=w522:errorcluster, "FP.State"=w520:T7)
            n232 = Not Equal?(x=w520, y=w518) -> (x != y?=w519:bool)
            n233 = case shown="True" w519 {
              tunnel: [w529 w530] -> w525
              tunnel: w522 -> [w528 w530]
              tunnel: w521 -> [w527 _]
              tunnel: w518 -> [w526 _]
              frame True {
                n234 = invoke class="VI" method="FP.Open"(reference=w527, error in=w528, "State"=w526) -> (error out=w529:errorcluster)  [unwired: 2 in, 4 out]
              }
              frame False {
              }
            }
          }
          frame "Maximize", "Maximized" {
            w531 = T7."Maximized" ("State")
            n235 = property class="VI"(reference=w537, error in=w536) -> (reference out=w534:refnum<vi>, error out=w535:errorcluster, "FP.State"=w533:T7)
            n236 = Not Equal?(x=w533, y=w531) -> (x != y?=w532:bool)
            n237 = case shown="True" w532 {
              tunnel: [w542 w543] -> w538
              tunnel: w535 -> [w541 w543]
              tunnel: w534 -> [w540 _]
              tunnel: w531 -> [w539 _]
              frame True {
                n238 = invoke class="VI" method="FP.Open"(reference=w540, error in=w541, "State"=w539) -> (error out=w542:errorcluster)  [unwired: 2 in, 4 out]
              }
              frame False {
              }
            }
          }
        }
        n239 = call <vilib>:"Add State(s) to Queue__jki_lib_state_machine.vi"("State(s) in (\"\")"=w478) -> ("States Out"=w477:string)  [unwired: 14 in]
      }
      frame "---------- Macro ----------" {
        # "Do not put any code in this frame.\n(It is a separator no-op. You can make a copy of this frame to create a new Macro frame)"
        n240 = call <vilib>:"Add State(s) to Queue__jki_lib_state_machine.vi"("State(s) in (\"\")"=w548) -> ("States Out"=w547:string)  [unwired: 14 in]
      }
      frame "Macro: Initialize" {
        # "Initialization Macro\n(This is called once, when the VI starts)"
        n241 = call <vilib>:"Add State(s) to Queue__jki_lib_state_machine.vi"("State(s) in Front (\"\")"="Data: Initialize\nInitialize Core Data\nEvents: Register\nUI: Initialize\nUI: Front Panel State >> Open\nActions: Get All Publishers IDs\nActions: Build Data\nUI: Populate Publishers", "State(s) in (\"\")"=w554) -> ("States Out"=w553:string)  [unwired: 13 in]
      }
      frame "Macro: Exit" {
        # "Exit Macro\n(This is called once, when the VI exits)"
        n242 = Unbundle By Name(w562) -> ("Core.Close Panel on Exit?"=w557:bool)
        n243 = call <vilib>:"Conditional State String__jki_lib_state_machine.vi"("Do State(s)?"=w557, "State"="UI: Front Panel State >> Close") -> ("State Out"=w556:string)  [unwired: 7 in]
        n244 = call <vilib>:"Add State(s) to Queue__jki_lib_state_machine.vi"("State(s) in (\"\")"=w556, "State(s) at Back (\"\")"="UI: Uninitialize\nData: Cleanup\nEvents: Unregister\nExit") -> ("States Out"=w560:string)  [unwired: 13 in]
        n245 = call <vilib>:"Add State(s) to Queue__jki_lib_state_machine.vi"("State(s) in Front (\"\")"=w560, "State(s) in (\"\")"=w564) -> ("States Out"=w563:string)  [unwired: 13 in]
      }
      frame "---------- Actions ----------" {
        n246 = call <vilib>:"Add State(s) to Queue__jki_lib_state_machine.vi"("State(s) in (\"\")"=w569) -> ("States Out"=w568:string)  [unwired: 14 in]
      }
      frame "Actions: Get All Publishers IDs" {
        n247 = Unbundle By Name(w573) -> ("manager_daemon"=w576:refnum<class "manager_daemon.lvclass">)
        n248 = call "get publishers.vi"("error in (no error)"=w575, "manager_daemon in"=w576) -> ("error out"=w571:errorcluster, "Publisher Map"=w574:T17)  [unwired: 7 in, 1 out]
        n249 = for {
          tunnel: w574 -> [w581] mode=indexing
          tunnel: [w580] -> w572 mode=indexing
          n250 = Unbundle By Name(w581) -> ("value.id"=w580:i32)
        }
        n251 = Bundle By Name(cluster=w573, "pub ids"=w572) -> (w570:T16)
        n252 = call <vilib>:"Add State(s) to Queue__jki_lib_state_machine.vi"("State(s) in (\"\")"=w579) -> ("States Out"=w578:string)  [unwired: 14 in]
      }
      frame "Actions: Zoom All" {
        # "Template Separator\n(You can make a copy of, or modify, this frame)"
        n253 = Unbundle By Name(w588) -> ("picture data.end date"=w583:timestamp, "picture data.start date"=w584:timestamp)
        n254 = property on="Plot Start" class="AbsTime (strict)"(error in=w587, "Val(Sgnl)"=w584) -> (error out=w586:errorcluster)  [unwired: 1 in, 1 out]
        n255 = property on="Plot End" class="AbsTime (strict)"(error in=w586, "Value"=w583) -> (error out=w585:errorcluster)  [unwired: 1 in, 1 out]
        n256 = call <vilib>:"Add State(s) to Queue__jki_lib_state_machine.vi"("State(s) in (\"\")"=w590) -> ("States Out"=w589:string)  [unwired: 14 in]
      }
      frame "Actions: Draw Grid" {
        n257 = property on="2D Picture" class="Pict"(error in=w599) -> (error out=w597:errorcluster, "Draw Area Size"=w598:T22, "Origin"=w591:T23)  [unwired: 1 in, 1 out]
        n258 = local read "Plot Start"() -> (w594:timestamp)
        n259 = local read "Plot End"() -> (w593:timestamp)
        n260 = call "create.grid.vi"("Point"=w591, "Draw Area Size"=w598, "Plot End"=w593, "Plot Start"=w594) -> ("picture"=w596:picture)  [unwired: 7 in]
        n261 = Bundle By Name(cluster=w600, "picture"=w596) -> (w595:T16)
        n262 = call <vilib>:"Add State(s) to Queue__jki_lib_state_machine.vi"("State(s) in (\"\")"=w602) -> ("States Out"=w601:string)  [unwired: 14 in]
      }
      frame "Actions: Display Cursor" {
        n263 = Unbundle By Name(w611) -> ("picture data.names"=w610:string[], "picture data.cells"=w609:T19, "cursor"=w608:T15)
        n264 = for {
          tunnel: w610 -> [w616] mode=indexing
          tunnel: w609 -> [w626] mode=indexing
          tunnel: w608 -> [w621]
          tunnel: [w616] -> w606
          tunnel: [w615] -> w607
          stop <- w615 stop-if-true
          n265 = Unbundle By Name(w621) -> ("Horizontal"=w620:i32, "Vertical"=w619:i32)
          n266 = Unbundle By Name(w626) -> ("right"=w625:i16, "left"=w624:i16, "bottom"=w623:i16, "top"=w622:i16)
          n267 = In Range and Coerce(upper limit=w625, x=w620, lower limit=w624) -> (In Range?=w618:bool)  [unwired: 1 out]
          n268 = In Range and Coerce(upper limit=w623, x=w619, lower limit=w622) -> (In Range?=w617:bool)  [unwired: 1 out]
          n269 = And(x=w618, y=w617) -> (x .and. y?=w615:bool)
        }
        n270 = Select(t=w606, s=w607, f="") -> (s? t:f=→"volume":string)
        n271 = call <vilib>:"Add State(s) to Queue__jki_lib_state_machine.vi"("State(s) in (\"\")"=w614) -> ("States Out"=w613:string)  [unwired: 14 in]
      }
      frame "Actions: Draw Picture" {
        n272 = property on="Legend" class="Clust (strict)"(error in=w629, "Visible"="Show Legend") -> (error out=w628:errorcluster)  [unwired: 1 in, 1 out]
        n273 = call <vilib>:"Add State(s) to Queue__jki_lib_state_machine.vi"("State(s) in (\"\")"=w633) -> ("States Out"=w632:string)  [unwired: 14 in]
      }
      frame "Actions: Build Data" {
        n274 = Unbundle By Name(w646) -> ("manager_daemon"=w647:refnum<class "manager_daemon.lvclass">, "filters.team filter"=w639:string[], "filters.char filter"=w638:string[], "filters.story filter"=w636:string[], "filters.concept filter"=w637:string[], "filters.Apply Filters"=w634:enum32{"AND", "OR"}, "pub ids"=w635:i32[])
        n275 = local read "Plot Start"() -> (w651:timestamp)
        n276 = local read "Plot End"() -> (w652:timestamp)
        n277 = Bundle(cluster=T10 {"Volume Type"={"Ongoing"=TRUE, "Limited Series"=TRUE, "Annuals"=TRUE, "One Shots"=TRUE, "Reference/Reprints"=TRUE, "Digital"=TRUE}, "team"=[], "characters"=[], "storyArcs"=[], "Plot End"=timestamp(0 s since 1904-01-01), "Plot Start"=timestamp(0 s since 1904-01-01), "title"=[], "colors"={"ongoing"=0, "Limited Series"=0, "Annuals"=0, "One Shots"=0, "Reprints"=0, "Digital"=0}, "concept"=[], "show all"=FALSE, "Search by Title"=enum."AND", "pub ids"=[]} ("selection filter"), "Volume Type"="Volume Type", "team"=w639, "characters"=w638, "storyArcs"=w636, "Plot End"=w652, "Plot Start"=w651, "title"="titles", "colors"="Legend", "concept"=w637, "show all"="Show All Comics", "Search by Title"=w634, "pub ids"=w635) -> (w641:T10)
        n278 = call "filter data.vi"("graph only (f)"=FALSE, "error in (no error)"=w644, "selection filter"=w641, "manager_daemon in"=w647) -> ("error out"=w645:errorcluster)  [unwired: 6 in, 1 out]
        n279 = call <vilib>:"Add State(s) to Queue__jki_lib_state_machine.vi"("State(s) in (\"\")"=w655) -> ("States Out"=w654:string)  [unwired: 14 in]
      }
      frame "Actions: Calculate Rows" {
        w657 = 16  # Row Height
        w658 = 32  # Row Height
        n280 = Unbundle By Name(w663) -> ("volume objects"=w666:cluster{"Array":T12[]}[])
        n281 = local read "Show/Hide Issues"() -> (w659:bool)
        n282 = Array Size(array=w666) -> (size(s)=w665:i32)
        n283 = Select(t=w658, s=w659, f=w657) -> (s? t:f=w656:i32)
        n284 = for {
          N: w665 -> [_]
          tunnel: T11 {"left"=0, "top"=0, "right"=0, "bottom"=0} ("rect") -> [w677]
          tunnel: [w676] -> w661 mode=indexing
          tunnel: w656 -> [w673]
          i -> [w675]
          n285 = Multiply(x=w673, y=w675) -> (x*y=w674:i32)
          n286 = Add(x=w674, y=w673) -> (x+y=w672:i32)
          n287 = Subtract(x=w672, y=2) -> (x-y=w670:i32)
          n288 = Bundle By Name(cluster=w677, "top"=w674, "bottom"=w670) -> (w676:T11)
        }
        n289 = Bundle By Name(cluster=w663, "rows"=w661) -> (w662:T16)
        n290 = call <vilib>:"Add State(s) to Queue__jki_lib_state_machine.vi"("State(s) in (\"\")"=w669) -> ("States Out"=w668:string)  [unwired: 14 in]
      }
      frame "Actions: Calculate Cells" {
        n291 = Unbundle By Name(w685) -> ("picture"=w686:picture, "volume objects"=w678:cluster{"Array":T12[]}[], "rows"=w690:T19)
        n292 = property on="2D Picture" class="Pict"() -> ("Draw Area Size"=w691:T22)  [unwired: 2 in, 2 out]
        n293 = Unbundle By Name(w691) -> ("Width"=w689:u32)
        n294 = local read "Plot Start"() -> (w688:timestamp)
        n295 = local read "Plot End"() -> (w687:timestamp)
        n296 = call "plot.volumes.vi"("plot end"=w687, "Show Issues"="Show/Hide Issues", "plot start"=w688, "picture in"=w686, "Width"=w689, "rows"=w690, "volume objects"=w678) -> ("names"=w681:string[], "cells"=w682:T19, "picture"=w683:picture)  [unwired: 2 in]
        "2D Picture" <- w683
        n297 = Bundle By Name(cluster=w685, "picture"=w683, "picture data.cells"=w682, "picture data.names"=w681) -> (w684:T16)
      }
    }
  }
